vi "Get I32.vi"(6 "LV Type":variant, 8 "error in (no error)":errorcluster, 9 "Data Type (default value)":i32, 10 "Offset":i32, 11 "JSON":string) -> (0 "error out":errorcluster, 1 "Number":i32, 2 "Offset past match":i32)   [LabVIEW 2019, in "JSONtext.lvlib"]
uses:
  JSONtext.lvlib
  String Subset.vi
  Parsing/Advance past Number.vi
  Format Error.vi
  Parsing/Parsing Error in converting to LabVIEW type.vi
  <vilib>/Utility/error.llb/Error Cluster From Error Code.vi
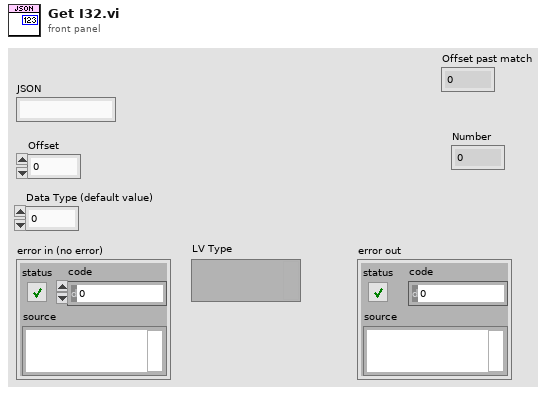
[diagram p1: front panel]
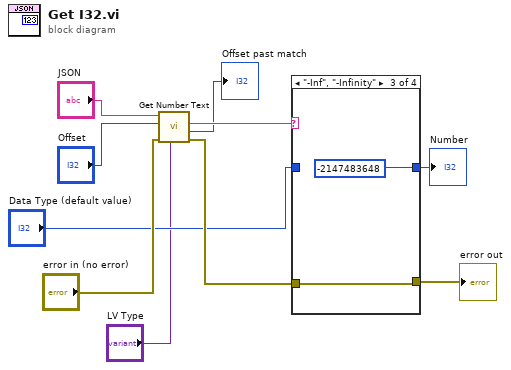
[diagram p0: block diagram]
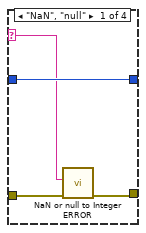
[diagram p2: hidden frame]
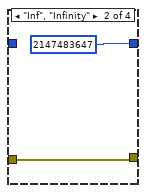
[diagram p3: hidden frame]
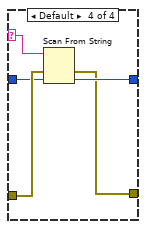
[diagram p4: hidden frame]
diagram:
  n1 = call "Get Number Text.vi"("LV Type"="LV Type", "error in (no error)"="error in (no error)", "Offset"="Offset", "JSON"="JSON") -> ("error out"=w7:errorcluster, "Offset past match"=→"Offset past match":i32, "Number Text"=w5:string)  [unwired: 4 in, 1 out]
  n2 = case shown="\"-Inf\", \"-Infinity\"" w5 {
    selector: w5 -> [w11 _ _ w19]
    tunnel: [w14 2147483647 ("default value 1") -2147483648 ("default value 1") w23] -> w4
    tunnel: w7 -> [w13 w15 w17 w22]
    tunnel: [w12 w15 w17 w21] -> w6
    tunnel: "Data Type (default value)" -> [w14 _ _ w20]
    frame "NaN", "null" {
      n3 = call "NaN or null to Integer ERROR.vi"("error in (no error)"=w13, "JSON NaN or null"=w11) -> ("error out"=w12:errorcluster)  [unwired: 9 in]
    }
    frame "Inf", "Infinity" {
    }
    frame "-Inf", "-Infinity" {
    }
    frame Default {
      n4 = Scan From String(input string=w19, error in=w22, default 1=w20) -> (error out=w21:errorcluster, output 1=w23:i32)  [unwired: 2 in, 2 out]
    }
  }
  "error out" <- w6
  "Number" <- w4
